vi "Cheesy Drive.vi"(5 "max queso power (1)":dbl=1.0, 6 "Quickturn":bool, 7 "Throttle Sensitivity":dbl=0.5, 8 "QuickTurn Sensitivty":dbl=0.7, 9 "Queso Arc Sensitivty":dbl=0.5, 10 "Wheel":dbl(slide) scale=-1.0..1.0, 11 "Throttle":dbl(slide) scale=-1.0..1.0) -> (2 "Right PWM":dbl, 3 "Left PWM":dbl)   [LabVIEW 2019]
panel:
  out "Waveform Chart 2":cluster{"left":dbl, "right":dbl}(graph)
  in  "alpha":dbl=0.1
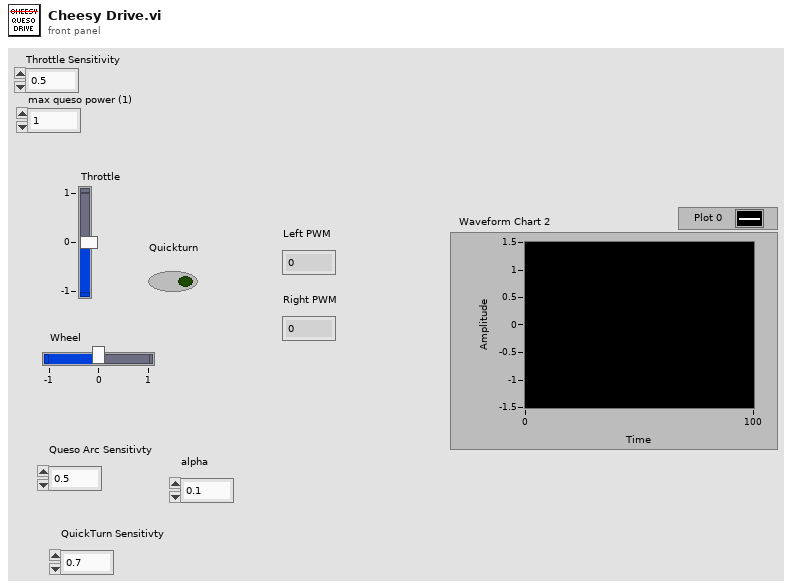
[diagram p1: front panel]
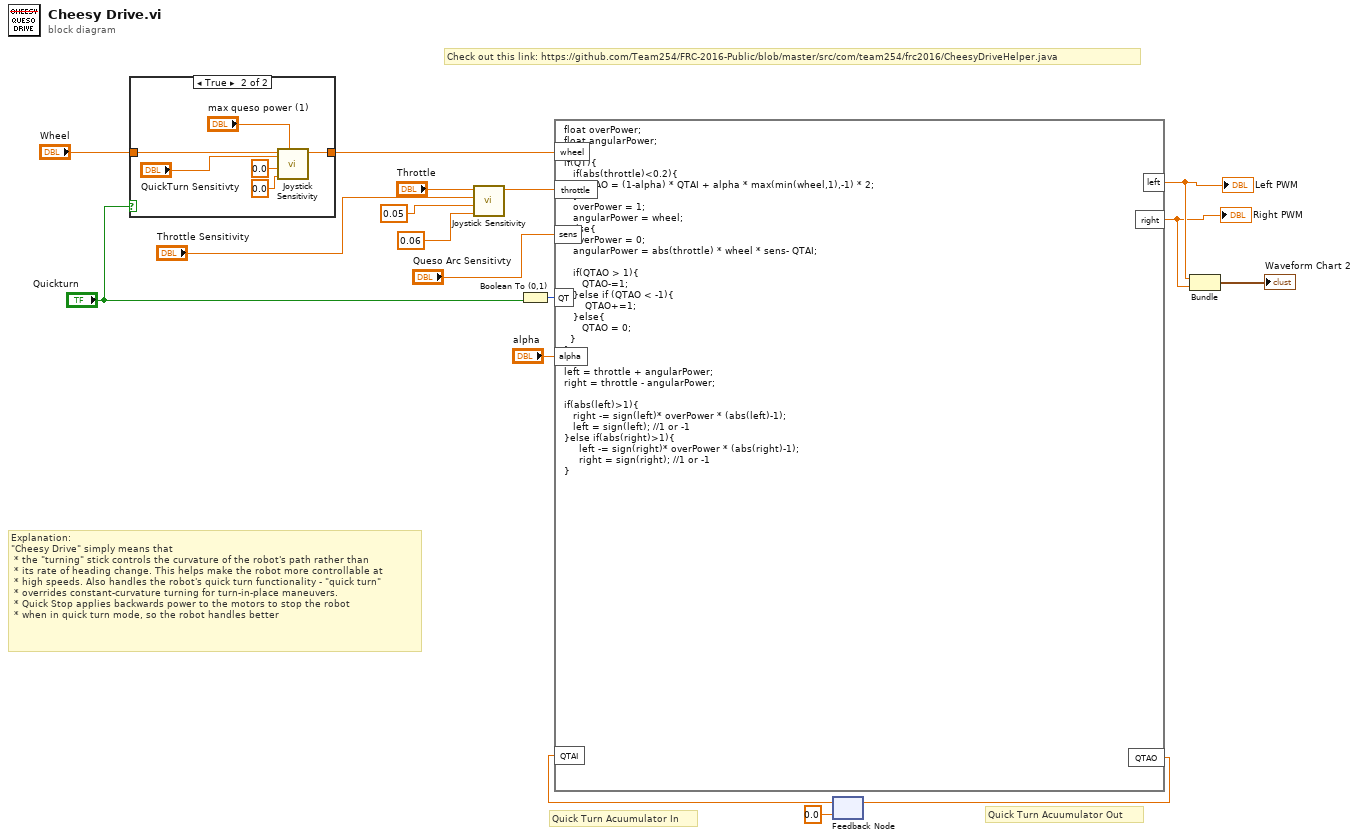
[diagram p0: block diagram]
diagram:
  # "Explanation:\n\"Cheesy Drive\" simply means that\n * the \"turning\" stick controls the curvature of the robot's path rather than\n * its rate of heading change. This helps make the robot more controllable at\n * high speeds. Also handles the robot's quick turn functionality - \"quick turn\"\n * overrides constant-curvature turning for turn-in-place maneuvers.\n * Quick Stop applies backwards power to the motors to stop the robot\n * when in quick turn mode, so the robot handles better"
  # "Quick Turn Acuumulator Out"
  # "Quick Turn Acuumulator In"
  # "Check out this link: https://github.com/Team254/FRC-2016-Public/blob/master/src/com/team254/frc2016/CheesyDriveHelper.java"
  n1 = case shown="True" "Quickturn" {
    tunnel: "Wheel" -> [w18 w24]
    tunnel: [w18 w23] -> w6
    frame False {
    }
    frame True {
      n2 = call "Joystick Sensitivity.vi"("max power (1)"="max queso power (1)", "joystick deadband"=0.0, "motor deadband (0.15)"=0.0, "sensitivity (0.5)"="QuickTurn Sensitivty", "x"=w24) -> ("y"=w23:dbl)  [unwired: 5 in, 1 out]
    }
  }
  n3 = call "Joystick Sensitivity.vi"("joystick deadband"=0.06, "motor deadband (0.15)"=0.05, "sensitivity (0.5)"="Throttle Sensitivity", "x"="Throttle") -> ("y"=w4:dbl)  [unwired: 6 in, 1 out]
  n4 = Boolean To (0,1)(Boolean="Quickturn") -> (0, 1=w15:i16)
  n5 = feedback #1(0.0 ("QTAccumulatorO")) -> (w13:dbl)
  n6 = formula code="float overPower;\nfloat angularPower;\n\nif(QT){\n   if(abs(throttle)<0.2){\n      QTAO = (1-alpha) * QTAI + alpha * max(min(wheel,1),-1) * 2;\n   }\n   overPower = 1;\n   angularPower = wheel;\n}else{\n   overPower = 0;\n   angularPower = abs(throttle) * wheel * sens- QTAI;\n\n   if(QTAO > 1){\n      QTAO-=1;\n   }else if (QTAO < -1){\n       QTAO+=1;\n   }else{\n      QTAO = 0;\n  }\n}\n\nleft = throttle + angularPower;\nright = throttle - angularPower;\n\nif(abs(left)>1){\n   right -= sign(left)* overPower * (abs(left)-1);\n   left = sign(left); //1 or -1\n}else if(abs(right)>1){\n     left -= sign(right)* overPower * (abs(right)-1);\n     right = sign(right); //1 or -1 \n}"("wheel"=w6, "throttle"=w4, "sens"="Queso Arc Sensitivty", "QT"=w15, "alpha"="alpha", "QTAI"=w13) -> ("left"=w10:dbl, "right"=w9:dbl, "QTAO"=w16:dbl)
  "Left PWM" <- w10
  "Right PWM" <- w9
  n7 = feedback-in #1(w16) -> ()
  n8 = Bundle("left"=w10, "right"=w9) -> (→"Waveform Chart 2":cluster{"left":dbl, "right":dbl})  [unwired: 1 in]
